vi "SysDef.Export.vi"(8 "error in (no error)":errorcluster, 11 "Node Ptr":T28 format="%.0x") -> (0 "error out":errorcluster, 3 "Configuration":T1={"Name"="", "Description"="", "Diagnostics Basic Configuraiton"={"CAN Interface"=enum."CAN0", "Baud Rate"=0, "Diagnostic Protocol"=enum."GMLAN", "Transport Protocol"=enum."ISO TP - Normal Mode", "Transmit ID"=0, "Receive ID"=0, "Transmit Extension"=0, "Receive Extension"=0, "Receive UUDT ID"=0, "Enable Stream"=TRUE, "VW TP Channel ID"=0, "Security"={"Source DLL Path"=path "", "Security Level"=1, "Target DLL Path"=path ""}, "Fill Frame"=FALSE, "Fill Byte"=255, "Termination"=FALSE}, "DID Outputs"={"Description"="", "Frames"=[]}, "DID Inputs"={"Description"="", "Frames"=[]}, "PID Outputs"={"Description"="", "Frames"=[]}, "PID Inputs"={"Description"="", "Frames"=[]}, "DPIDs"={"Description"="", "DPIDs"=[]}, "DTC"={"Description"="", "DTC descriptor"={"DTC Byte Length"=2, "Status Byte Length"=1, "Add Data Byte Length"=1, "Byte Order"=enum."Motorola"}, "DTC Control"={"Description"="", "Signals"=[]}}, "NI 986x Support"={"Enable"=FALSE, "RIO Device"=0, "Bitfile"=path ""}, "Commands"={"Description"=""}, "Status"={"Description"=""}, "IO Controls"={"Description"="", "IO Control Array"=[]}, "Routines"={"Description"="", "Routine Array"=[]}, "Memory Outputs"={"Description"="", "Frames"=[]}, "Memory Inputs"={"Description"="", "Frames"=[]}, "User Defined"={"Description"="", "Groups"=[]}} {"DID Outputs"."Frames"."Signals"."Byte Order" items=["Little Endian", "Big Endian"]; "DID Outputs"."Frames"."Signals"."Data Type" items=["Signed", "Unsigned", "IEEE Float"]; "Memory Inputs"."Frames"."Signals"."Byte Order" items=["Little Endian", "Big Endian"]; "Memory Inputs"."Frames"."Signals"."Data Type" items=["Signed", "Unsigned", "IEEE Float"]; "Memory Outputs"."Frames"."Signals"."Byte Order" items=["Little Endian", "Big Endian"]; "Memory Outputs"."Frames"."Signals"."Data Type" items=["Signed", "Unsigned", "IEEE Float"]; "Routines"."Routine Array"."Stop Parameters"."Response"."Byte Order" items=["Little Endian", "Big Endian"]; "Routines"."Routine Array"."Stop Parameters"."Response"."Data Type" items=["Signed", "Unsigned", "IEEE Float"]; "Routines"."Routine Array"."Stop Parameters"."Cmd"."Byte Order" items=["Little Endian", "Big Endian"]; "Routines"."Routine Array"."Stop Parameters"."Cmd"."Data Type" items=["Signed", "Unsigned", "IEEE Float"]; "Routines"."Routine Array"."Request Parameters"."Response"."Byte Order" items=["Little Endian", "Big Endian"]; "Routines"."Routine Array"."Request Parameters"."Response"."Data Type" items=["Signed", "Unsigned", "IEEE Float"]; "Routines"."Routine Array"."Request Parameters"."Cmd"."Byte Order" items=["Little Endian", "Big Endian"]; "Routines"."Routine Array"."Request Parameters"."Cmd"."Data Type" items=["Signed", "Unsigned", "IEEE Float"]; "Routines"."Routine Array"."Start Parameters"."Response"."Byte Order" items=["Little Endian", "Big Endian"]; "Routines"."Routine Array"."Start Parameters"."Response"."Data Type" items=["Signed", "Unsigned", "IEEE Float"]; "Routines"."Routine Array"."Start Parameters"."Cmd"."Byte Order" items=["Little Endian", "Big Endian"]; "Routines"."Routine Array"."Start Parameters"."Cmd"."Data Type" items=["Signed", "Unsigned", "IEEE Float"]; "IO Controls"."IO Control Array"."Signals"."Response"."Byte Order" items=["Little Endian", "Big Endian"]; "IO Controls"."IO Control Array"."Signals"."Response"."Data Type" items=["Signed", "Unsigned", "IEEE Float"]; "IO Controls"."IO Control Array"."Signals"."Cmd"."Byte Order" items=["Little Endian", "Big Endian"]; "IO Controls"."IO Control Array"."Signals"."Cmd"."Data Type" items=["Signed", "Unsigned", "IEEE Float"]; "DTC"."DTC Control"."Signals"."Byte Order" items=["Little Endian", "Big Endian"]; "DTC"."DTC Control"."Signals"."Data Type" items=["Signed", "Unsigned", "IEEE Float"]; "Diagnostics Basic Configuraiton"."Fill Byte" format="%.0x"; "Diagnostics Basic Configuraiton"."VW TP Channel ID" format="%.0x"; "Diagnostics Basic Configuraiton"."Receive UUDT ID" format="%.0x"; "Diagnostics Basic Configuraiton"."Receive Extension" format="%.0x"; "Diagnostics Basic Configuraiton"."Transmit Extension" format="%.0x"; "Diagnostics Basic Configuraiton"."Receive ID" format="%.0x"; "Diagnostics Basic Configuraiton"."Transmit ID" format="%.0x"; "DID Inputs"."Frames"."Signals"."Byte Order" items=["Little Endian", "Big Endian"]; "DID Inputs"."Frames"."Signals"."Data Type" items=["Signed", "Unsigned", "IEEE Float"]; "PID Inputs"."Frames"."Signals"."Byte Order" items=["Little Endian", "Big Endian"]; "PID Inputs"."Frames"."Signals"."Data Type" items=["Signed", "Unsigned", "IEEE Float"]; "PID Outputs"."Frames"."Signals"."Byte Order" items=["Little Endian", "Big Endian"]; "PID Outputs"."Frames"."Signals"."Data Type" items=["Signed", "Unsigned", "IEEE Float"]})   [LabVIEW 2015, in "Diagnostics Addon System Explorer.lvlib"]
uses:
  Diagnostics Addon System Explorer.lvlib
  <vilib>/NI Veristand/Custom Device API/Custom Device Item Ref.ctl
  Types/SysDef.Export.ctl
  Shared/Types/CAN.ctl
  Shared/Types/CAN.Interface.ctl
  Shared/Types/Protocol.ctl
  Shared/Types/Transport.ctl
  Shared/Types/Security.ctl
  Types/Frames.Export.ctl
  Types/Frame.Export.ctl
  Shared/Types/Signal.ctl
  Types/DPIDs.Export.ctl
  Types/DPID.Export.ctl
  Shared/Types/DPID.ctl
  Shared/Types/DPID.Rate.ctl
  Types/DTC.Export.ctl
  Shared/Types/DTCDescriptor.ctl
  Types/DTCControl.Export.ctl
  Shared/Types/986x.ctl
  Types/Command.Export.ctl
  Types/Status.Export.ctl
  Types/IOControls.Export.ctl
  Types/IO.Export.ctl
  Types/CmdResp.Export.ctl
  Types/Routines.Export.ctl
  Types/Routine.Export.ctl
  Types/UserDefined.Export.ctl
  Types/UserDefined.Group.Export.ctl
  Types/UserDefined.Group.Message.Export.ctl
  Types/FG.Action.ctl
  FileDependency.Create.vi
  Frame.Export.vi
  DPID.FG.vi
  Frame.Convert.Name.vi
  DTCDescriptor.FG.vi
  Routine.Export.vi
  Signals.Get.vi
  Type.FG.vi
  IO.Export.vi
  UserDefined.Group.Export.vi
  ID.FG.vi
  CmdResp.Export.vi
  Signal.FG.vi
  <vilib>/NI Veristand/Custom Device Tools/Custom Device Utility Library/NI VeriStand - Search for Item by GUID.vi
  <vilib>/NI Veristand/Custom Device API/NI VeriStand - Get Item Property.vi
  <vilib>/NI Veristand/Custom Device API/Get Item Property (U32).vi
  <vilib>/NI Veristand/Custom Device API/NI VeriStand - Set Item Property.vi
  <vilib>/NI Veristand/Custom Device API/Set Item Property (U32).vi
  Shared/SubVIs/Constants.vi
  <vilib>/NI Veristand/Custom Device API/NI VeriStand - Get Custom Device Channel Data.vi
  <vilib>/NI Veristand/Custom Device API/Get Item Property (String).vi
  <vilib>/NI Veristand/Custom Device API/Get Item Property (Double).vi
  <vilib>/NI Veristand/Custom Device API/Set Item Property (String).vi
  <vilib>/NI Veristand/Custom Device API/Set Item Property (Double).vi
  <vilib>/NI Veristand/Custom Device API/NI VeriStand - Get Item Children.vi
  <vilib>/NI Veristand/Custom Device Tools/Custom Device Utility Library/NI VeriStand - Search for All Items by GUID.vi
  <vilib>/NI Veristand/Custom Device API/Get Item Property (I32).vi
  <vilib>/NI Veristand/Custom Device API/Set Item Property (I32).vi
  <vilib>/NI Veristand/Custom Device API/Get Item Property (U32 Array).vi
  <vilib>/NI Veristand/Custom Device API/Set Item Property (U32 Array).vi
  <vilib>/NI Veristand/Custom Device API/Get Item Property (Dependent File).vi
  <vilib>/NI Veristand/Custom Device API/Get Item Property (U16).vi
  <vilib>/NI Veristand/Custom Device API/Get Item Property (Boolean).vi
  <vilib>/NI Veristand/Custom Device API/Set Item Property (Boolean).vi
  <vilib>/NI Veristand/Custom Device API/NI VeriStand - Remove Item Property.vi
  <vilib>/NI Veristand/Custom Device API/Set Item Property (Dependent File).vi
  <vilib>/Utility/MD5Checksum.llb/MD5Checksum File.vi
  FileDependency.Get.Target Path.vi
  <vilib>/NI Veristand/Custom Device API/Custom Device API.lvlib
  Shared/Diagnostics Addon Shared.lvlib
  <vilib>/NI Veristand/Custom Device Tools/Custom Device Utility Library/Custom Device Utility Library.lvlib
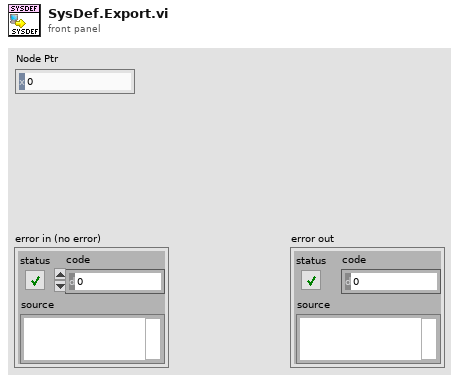
[diagram p1: front panel]
types:
  T1 = typedef "Diagnostics Addon System Explorer.lvlib/SysDef.Export.ctl" = cluster{"Name":string, "Description":string, "Diagnostics Basic Configuraiton":T2, "DID Outputs":T7, "DID Inputs":T7, "PID Outputs":T7, "PID Inputs":T7, "DPIDs":T10, "DTC":T14, "NI 986x Support":T17, "Commands":T18, "Status":T19, "IO Controls":T20, "Routines":T23, "Memory Outputs":T7, "Memory Inputs":T7, "User Defined":T25}
  T2 = typedef "Diagnostics Addon Shared.lvlib/CAN.ctl" = cluster{"CAN Interface":T3, "Baud Rate":u32, "Diagnostic Protocol":T4, "Transport Protocol":T5, "Transmit ID":u32, "Receive ID":u32, "Transmit Extension":u8, "Receive Extension":u8, "Receive UUDT ID":u32, "Enable Stream":bool, "VW TP Channel ID":u32, "Security":T6, "Fill Frame":bool, "Fill Byte":u8, "Termination":bool}
  T3 = typedef "Diagnostics Addon Shared.lvlib/CAN.Interface.ctl" = enum16{"CAN0", "CAN1", "CAN2", "CAN3", "CAN4", "CAN5", "CAN6", "CAN7", "CAN8", "CAN9", "CAN10", "CAN11", "CAN12", "CAN13", "CAN14", "CAN15", "CAN16", "CAN17", "CAN18", "CAN19", "CAN20", "CAN21", "CAN22", "CAN23", "CAN24", "CAN25", "CAN26", "CAN27", "CAN28", "CAN29", "CAN30", "CAN31", "CAN32", "CAN33", "CAN34", "CAN35", "CAN36", "CAN37", "CAN38", "CAN39", "CAN40", "CAN41", "CAN42", "CAN43", "CAN44", "CAN45", "CAN46", "CAN47", "CAN48", "CAN49", "CAN50", "CAN51", "CAN52", "CAN53", "CAN54", "CAN55", "CAN56", "CAN57", "CAN58", "CAN59", "CAN60", "CAN61", "CAN62", "CAN63", "CAN 256 (Virtual)", "CAN 257 (Virtual)"}
  T4 = typedef "Diagnostics Addon Shared.lvlib/Protocol.ctl" = enum16{"GMLAN", "KWP-2000", "UDS"}
  T5 = typedef "Diagnostics Addon Shared.lvlib/Transport.ctl" = enum16{"ISO TP - Normal Mode", "ISO TP - Mixed Mode", "VW TP 2.0", "Diagnostics on IP"}
  T6 = typedef "Diagnostics Addon Shared.lvlib/Security.ctl" = cluster{"Source DLL Path":path, "Security Level":u8, "Target DLL Path":path}
  T7 = typedef "Diagnostics Addon System Explorer.lvlib/Frames.Export.ctl" = cluster{"Description":string, "Frames":T8[]}
  T8 = typedef "Diagnostics Addon System Explorer.lvlib/Frame.Export.ctl" = cluster{"Name":string, "Description":string, "ID":u32, "Signals":T9[]}
  T9 = typedef "Diagnostics Addon Shared.lvlib/Signal.ctl" = cluster{"Start Bit":u8, "Length":u8, "Scaling Factor":dbl, "Scaling Offset":dbl, "Minimum":dbl, "Maximum":dbl, "Data Type":u32, "Byte Order":u32, "Default Value":dbl, "Name":string, "Units":string, "Description":string}
  T10 = typedef "Diagnostics Addon System Explorer.lvlib/DPIDs.Export.ctl" = cluster{"Description":string, "DPIDs":T11[]}
  T11 = typedef "Diagnostics Addon System Explorer.lvlib/DPID.Export.ctl" = cluster{"Name":string, "Description":string, "DPID":T12}
  T12 = typedef "Diagnostics Addon Shared.lvlib/DPID.ctl" = cluster{"DPID ID":u8, "Speed":T13, "PIDs":u16[]}
  T13 = typedef "Diagnostics Addon Shared.lvlib/DPID.Rate.ctl" = enum16{"Slow", "Medium", "Fast"}
  T14 = typedef "Diagnostics Addon System Explorer.lvlib/DTC.Export.ctl" = cluster{"Description":string, "DTC descriptor":T15, "DTC Control":T16}
  T15 = typedef "Diagnostics Addon Shared.lvlib/DTCDescriptor.ctl" = cluster{"DTC Byte Length":i32, "Status Byte Length":i32, "Add Data Byte Length":i32, "Byte Order":enum16{"Motorola", "Intel"}}
  T16 = typedef "Diagnostics Addon System Explorer.lvlib/DTCControl.Export.ctl" = cluster{"Description":string, "Signals":T9[]}
  T17 = typedef "Diagnostics Addon Shared.lvlib/986x.ctl" = cluster{"Enable":bool, "RIO Device":u16, "Bitfile":path}
  T18 = typedef "Diagnostics Addon System Explorer.lvlib/Command.Export.ctl" = cluster{"Description":string}
  T19 = typedef "Diagnostics Addon System Explorer.lvlib/Status.Export.ctl" = cluster{"Description":string}
  T20 = typedef "Diagnostics Addon System Explorer.lvlib/IOControls.Export.ctl" = cluster{"Description":string, "IO Control Array":T21[]}
  T21 = typedef "Diagnostics Addon System Explorer.lvlib/IO.Export.ctl" = cluster{"Name":string, "Description":string, "ID":u16, "Signals":T22}
  T22 = typedef "Diagnostics Addon System Explorer.lvlib/CmdResp.Export.ctl" = cluster{"Cmd":T9[], "Response":T9[]}
  T23 = typedef "Diagnostics Addon System Explorer.lvlib/Routines.Export.ctl" = cluster{"Description":string, "Routine Array":T24[]}
  T24 = typedef "Diagnostics Addon System Explorer.lvlib/Routine.Export.ctl" = cluster{"Name":string, "Description":string, "ID":u16, "Start Parameters":T22, "Request Parameters":T22, "Stop Parameters":T22}
  T25 = typedef "Diagnostics Addon System Explorer.lvlib/UserDefined.Export.ctl" = cluster{"Description":string, "Groups":T26[]}
  T26 = typedef "Diagnostics Addon System Explorer.lvlib/UserDefined.Group.Export.ctl" = cluster{"Name":string, "Description":string, "Messages":T27[]}
  T27 = typedef "Diagnostics Addon System Explorer.lvlib/UserDefined.Group.Message.Export.ctl" = cluster{"Name":string, "Description":string, "Signals":T22}
  T28 = typedef "Custom Device API.lvlib/Custom Device Item Ref.ctl" = u64
  T29 = typedef "Diagnostics Addon System Explorer.lvlib/FG.Action.ctl" = enum16{"Get", "Set"}
  T30 = typedef "Custom Device API.lvlib/Custom Device Item Info.ctl" = cluster{"Name":string, "Is Channel":bool, "GUID":string, "Is Waveform":bool}
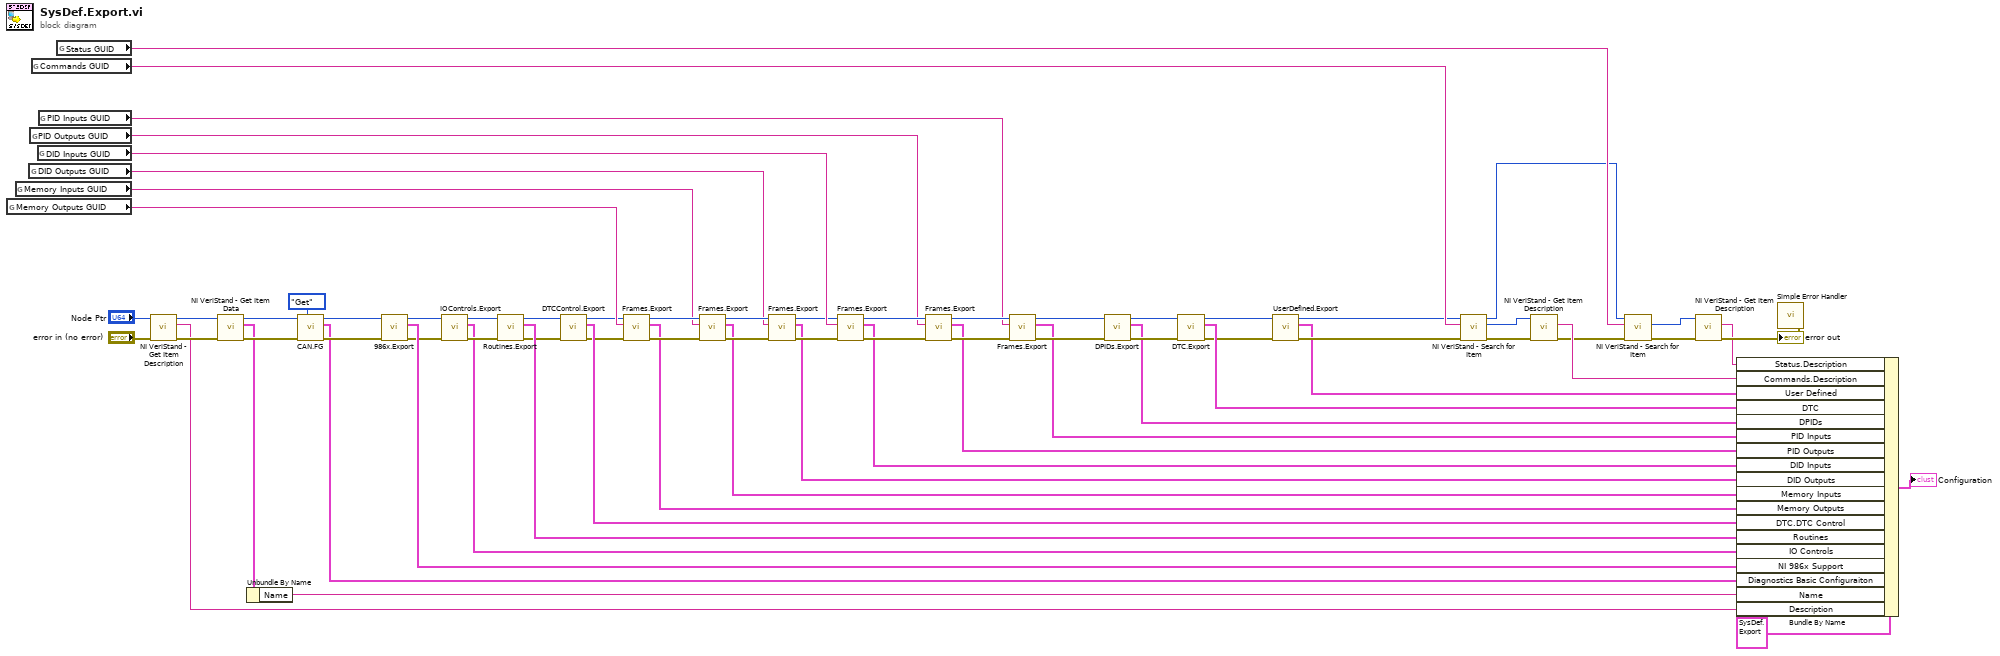
[diagram p0: block diagram]
diagram:
  n1 = global read "Constants.vi" "Memory Outputs GUID"() -> (w20:string)
  n2 = global read "Constants.vi" "Memory Inputs GUID"() -> (w21:string)
  n3 = global read "Constants.vi" "DID Outputs GUID"() -> (w22:string)
  n4 = global read "Constants.vi" "PID Outputs GUID"() -> (w58:string)
  n5 = global read "Constants.vi" "Commands GUID"() -> (w39:string)
  n6 = global read "Constants.vi" "DID Inputs GUID"() -> (w63:string)
  n7 = global read "Constants.vi" "PID Inputs GUID"() -> (w57:string)
  n8 = global read "Constants.vi" "Status GUID"() -> (w31:string)
  n9 = call <vilib>:"NI VeriStand - Get Item Description.vi"("error in (no error)"="error in (no error)", "Item Ref in"="Node Ptr") -> ("error out"=w70:errorcluster, "Description"=w55:string, "Item Ref out"=w71:T28)  [unwired: 7 out]
  n10 = call <vilib>:"NI VeriStand - Get Item Data.vi"("error in (no error)"=w70, "Item Ref in"=w71) -> ("error out"=w68:errorcluster, "Item Info"=w54:T30, "Item Ref out"=w69:T28)  [unwired: 7 out]
  n11 = Unbundle By Name(w54) -> ("Name"=w53:string)
  n12 = call "CAN.FG.vi"("Action"=FG.Action."Get", "error in (no error)"=w68, "Device Item Ref in"=w69) -> ("error out"=w66:errorcluster, "Diagnostics Basic Configuraiton"=w47:T2, "Device Item Ref out"=w67:T28)  [unwired: 6 in]
  n13 = call "986x.Export.vi"("error in (no error)"=w66, "Device Item Ref in"=w67) -> ("error out"=w19:errorcluster, "986x Support"=w40:T17, "Item Ref out"=w18:T28)  [unwired: 7 in]
  n14 = call "IOControls.Export.vi"("error in (no error)"=w19, "Item Ref in"=w18) -> ("error out"=w17:errorcluster, "IO Controls"=w15:T20, "Section Ref out"=w16:T28)  [unwired: 7 in]
  n15 = call "Routines.Export.vi"("error in (no error)"=w17, "Item Ref in"=w16) -> ("error out"=w9:errorcluster, "Routines"=w14:T23, "Section Ref out"=w10:T28)  [unwired: 7 in]
  n16 = call "DTCControl.Export.vi"("error in (no error)"=w9, "Section Ref in"=w10) -> ("error out"=w6:errorcluster, "DTCControl"=w7:T16, "Section Ref out"=w8:T28)  [unwired: 7 in]
  n17 = call "Frames.Export.vi"("error in (no error)"=w6, "GUID"=w20, "Item Ref in"=w8) -> ("error out"=w23:errorcluster, "Section"=w12:T7, "Section Ref out"=w26:T28)  [unwired: 6 in]
  n18 = call "Frames.Export.vi"("error in (no error)"=w23, "GUID"=w21, "Item Ref in"=w26) -> ("error out"=w24:errorcluster, "Section"=w13:T7, "Section Ref out"=w25:T28)  [unwired: 6 in]
  n19 = call "Frames.Export.vi"("error in (no error)"=w24, "GUID"=w22, "Item Ref in"=w25) -> ("error out"=w27:errorcluster, "Section"=w11:T7, "Section Ref out"=w28:T28)  [unwired: 6 in]
  n20 = call "Frames.Export.vi"("error in (no error)"=w27, "GUID"=w63, "Item Ref in"=w28) -> ("error out"=w59:errorcluster, "Section"=w52:T7, "Section Ref out"=w61:T28)  [unwired: 6 in]
  n21 = call "Frames.Export.vi"("error in (no error)"=w59, "GUID"=w58, "Item Ref in"=w61) -> ("error out"=w62:errorcluster, "Section"=w51:T7, "Section Ref out"=w60:T28)  [unwired: 6 in]
  n22 = call "Frames.Export.vi"("error in (no error)"=w62, "GUID"=w57, "Item Ref in"=w60) -> ("error out"=w56:errorcluster, "Section"=w50:T7, "Section Ref out"=w41:T28)  [unwired: 6 in]
  n23 = call "DPIDs.Export.vi"("error in (no error)"=w56, "Section Ref in"=w41) -> ("error out"=w49:errorcluster, "DPIDs"=w44:T10, "Section Ref out"=w45:T28)  [unwired: 7 in]
  n24 = call "DTC.Export.vi"("error in (no error)"=w49, "Section Ref in"=w45) -> ("error out"=w4:errorcluster, "DTC"=w43:T14, "Section Ref out"=w5:T28)  [unwired: 7 in]
  n25 = call "UserDefined.Export.vi"("error in (no error)"=w4, "Item Ref in"=w5) -> ("error out"=w2:errorcluster, "User Defined"=w1:T25, "Section Ref out"=w3:T28)  [unwired: 7 in]
  n26 = call-poly <vilib>:"NI VeriStand - Search for Item.vi"("error in"=w2, "Item GUID"=w39, "Section Ref in"=w3) -> ("error out"=w37:errorcluster, "Item Ref"=w38:T28, "Section Ref out"=w30:T28)  [unwired: 5 in, 1 out]
  n27 = call <vilib>:"NI VeriStand - Get Item Description.vi"("error in (no error)"=w37, "Item Ref in"=w38) -> ("error out"=w33:errorcluster, "Description"=w36:string)  [unwired: 8 out]
  n28 = call-poly <vilib>:"NI VeriStand - Search for Item.vi"("error in"=w33, "Item GUID"=w31, "Section Ref in"=w30) -> ("error out"=w35:errorcluster, "Item Ref"=w34:T28)  [unwired: 5 in, 2 out]
  n29 = call <vilib>:"NI VeriStand - Get Item Description.vi"("error in (no error)"=w35, "Item Ref in"=w34) -> ("error out"=w32:errorcluster, "Description"=w29:string)  [unwired: 8 out]
  "error out" <- w32
  n30 = Bundle By Name(cluster=T1 {"Name"="", "Description"="", "Diagnostics Basic Configuraiton"={"CAN Interface"=enum."CAN0", "Baud Rate"=0, "Diagnostic Protocol"=enum."GMLAN", "Transport Protocol"=enum."ISO TP - Normal Mode", "Transmit ID"=0, "Receive ID"=0, "Transmit Extension"=0, "Receive Extension"=0, "Receive UUDT ID"=0, "Enable Stream"=FALSE, "VW TP Channel ID"=0, "Security"={"Source DLL Path"=path "", "Security Level"=1, "Target DLL Path"=path ""}, "Fill Frame"=FALSE, "Fill Byte"=255, "Termination"=FALSE}, "DID Outputs"={"Description"="", "Frames"=[]}, "DID Inputs"={"Description"="", "Frames"=[]}, "PID Outputs"={"Description"="", "Frames"=[]}, "PID Inputs"={"Description"="", "Frames"=[]}, "DPIDs"={"Description"="", "DPIDs"=[]}, "DTC"={"Description"="", "DTC descriptor"={"DTC Byte Length"=0, "Status Byte Length"=0, "Add Data Byte Length"=0, "Byte Order"=enum."Motorola"}, "DTC Control"={"Description"="", "Signals"=[]}}, "NI 986x Support"={"Enable"=FALSE, "RIO Device"=0, "Bitfile"=path ""}, "Commands"={"Description"=""}, "Status"={"Description"=""}, "IO Controls"={"Description"="", "IO Control Array"=[]}, "Routines"={"Description"="", "Routine Array"=[]}, "Memory Outputs"={"Description"="", "Frames"=[]}, "Memory Inputs"={"Description"="", "Frames"=[]}, "User Defined"={"Description"="", "Groups"=[]}} ("Configuration"), "Status.Description"=w29, "Commands.Description"=w36, "User Defined"=w1, "DTC"=w43, "DPIDs"=w44, "PID Inputs"=w50, "PID Outputs"=w51, "DID Inputs"=w52, "DID Outputs"=w11, "Memory Inputs"=w13, "Memory Outputs"=w12, "DTC.DTC Control"=w7, "Routines"=w14, "IO Controls"=w15, "NI 986x Support"=w40, "Diagnostics Basic Configuraiton"=w47, "Name"=w53, "Description"=w55) -> (→"Configuration":T1)
  n31 = call <vilib>:"Simple Error Handler.vi"("error in (no error)"=w32) -> ()  [unwired: 4 in, 5 out]
